vi "get_data.vi"(0 "HGF_DIMService":refnum<class "HGF_DIMService.lvclass">, 5 "error in (no error)":errorcluster) -> (14 "dup HGF_DIMService":refnum<class "HGF_DIMService.lvclass">, 16 "serviceID":i32, 17 "data":string, 18 "quality":i32, 19 "error out":errorcluster)   [LabVIEW 2012, in "HGF_DIM.lvlib" / "HGF_DIMService.lvclass"]
uses:
  HGF_DIMService.lvclass
  HGF_DIMService.lvclass/HGF_DIMService.ctl
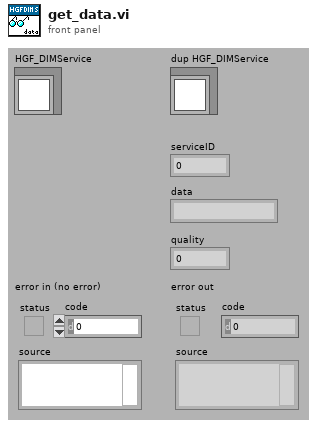
[diagram p1: front panel]
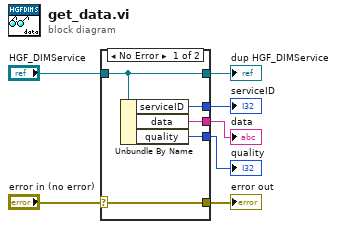
[diagram p0: block diagram]
diagram:
  n1 = case shown="No Error" "error in (no error)" {
    selector: "error in (no error)" -> [w12 w13]
    tunnel: [w12 w13] -> w6
    tunnel: [w11 w14] -> w4
    tunnel: "HGF_DIMService" -> [w11 w14]
    tunnel: [w10 _] -> w3
    tunnel: [w9 _] -> w2
    tunnel: [w8 _] -> w1
    frame No Error {
      n2 = Unbundle By Name(w11) -> ("serviceID"=w10:i32, "data"=w9:string, "quality"=w8:i32)
    }
    frame Error {
    }
  }
  "error out" <- w6
  "dup HGF_DIMService" <- w4
  "serviceID" <- w3
  "data" <- w2
  "quality" <- w1
